vi "Number to Match SB.vi"() -> ()   [LabVIEW 2019]
panel:
  in  "Cease":bool
  out "Iterations":i32
  in  "Number to Match":i32 min=0 max=100
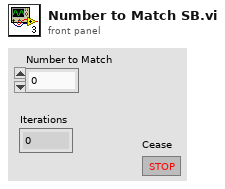
[diagram p1: front panel]
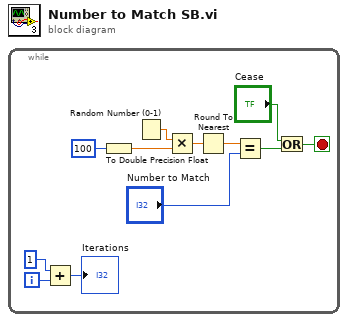
[diagram p0: block diagram]
diagram:
  n1 = while {
    i -> [w8]
    stop <- w5 stop-if-true
    n2 = Add(x=1, y=w8) -> (x+y=→"Iterations":i32)
    n3 = To Double Precision Float(number=100) -> (double precision float=w10:dbl)
    n4 = Random Number (0-1)() -> (number: 0 to 1=w12:dbl)
    n5 = Multiply(x=w12, y=w10) -> (x*y=w2:dbl)
    n6 = Round To Nearest(number=w2) -> (nearest integer value=w1:dbl)
    n7 = Equal?(x=w1, y="Number to Match") -> (x = y?=w4:bool)
    n8 = Or(x="Cease", y=w4) -> (x .or. y?=w5:bool)
  }
